vi "DAC Init Results.vi"(8 "error in":errorcluster, 9 "Log Details?":bool, 10 "tdms file":refnum<k34>, 11 "DAC Vacum Valve in":refnum<class "DAC Vacum Valve.lvclass">) -> (0 "error out":errorcluster, 2 "tdms file out":refnum<k34>)   [LabVIEW 2019, in "DAC.lvlib" / "DAC Vacum Valve.lvclass"]
uses:
  DAC Vacum Valve.lvclass
  C:/Users/krio/Documents/LV_Projects/test-stand/App/DAC/DAC.lvclass
  DAC.lvclass/DAC.ctl
  DAC Vacum Valve.lvclass/DAC Vacum Valve.ctl
  DAC.lvclass
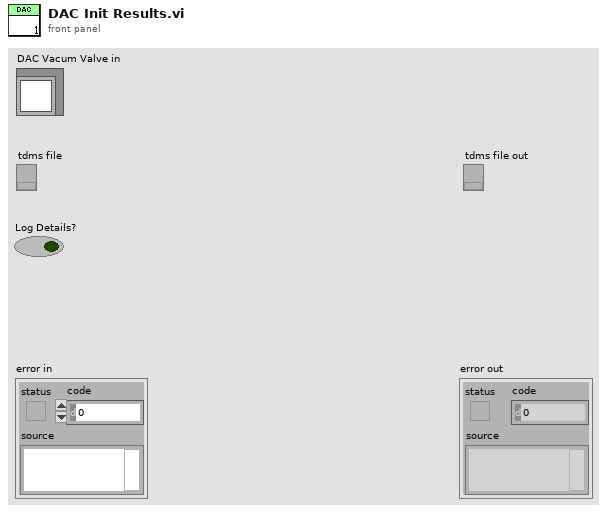
[diagram p1: front panel]
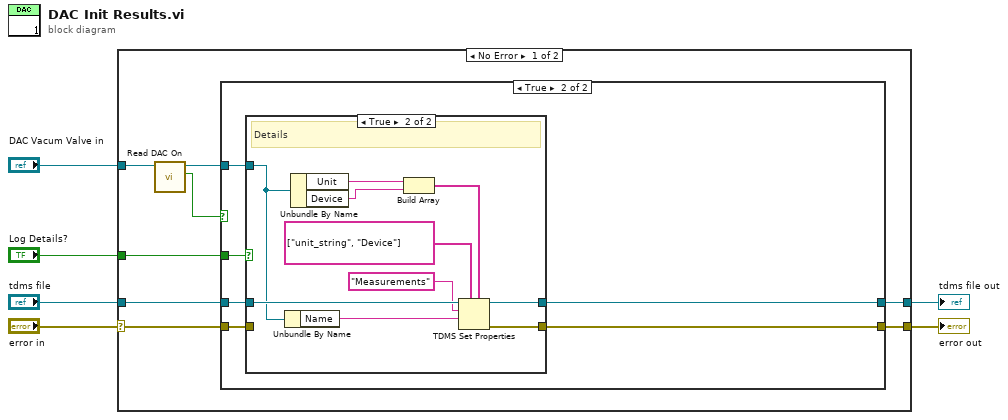
[diagram p0: block diagram]
diagram:
  n1 = case shown="No Error" "error in" {
    selector: "error in" -> [w10 w36]
    tunnel: [w7 w36] -> w6
    tunnel: "DAC Vacum Valve in" -> [w14 _]
    tunnel: "tdms file" -> [w11 w35]
    tunnel: [w8 w35] -> w5
    tunnel: "Log Details?" -> [w9 _]
    frame No Error {
      n2 = call "Read DAC On.vi"("DAC in"=w14) -> ("DAC On"=w12:bool, "DAC out"=w13:refnum<class "DAC Vacum Valve.lvclass">)  [unwired: 8 in, 1 out]
      n3 = case shown="True" w12 {
        tunnel: w11 -> [w15 w22]
        tunnel: [w15 w19] -> w8
        tunnel: [w16 w18] -> w7
        tunnel: w13 -> [_ w21]
        tunnel: w10 -> [w16 w17]
        tunnel: w9 -> [_ w20]
        frame False {
        }
        frame True {
          n4 = case shown="True" w20 {
            tunnel: w22 -> [w24 w34]
            tunnel: [w24 w29] -> w19
            tunnel: [w23 w28] -> w18
            tunnel: w21 -> [_ w25]
            tunnel: w17 -> [w23 _]
            frame False {
            }
            frame True {
              # "Details"
              n5 = Unbundle By Name(w25) -> ("Name"=w27:string)
              n6 = Unbundle By Name(w25) -> ("Unit"=w31:string, "Device"=w26:string)
              n7 = Build Array(w31, w26) -> (w30:string[])
              n8 = TDMS Set Properties(5:w30, 7:string[] ["unit_string", "Device"] ("property names"), 9:w27, 10:"Measurements" ("group name in (Untitled)"), 11:w34) -> (0:w28:errorcluster, 3:w29:refnum<k34>)  [unwired: 1 in, 2 out]
            }
          }
        }
      }
    }
    frame Error {
    }
  }
  "error out" <- w6
  "tdms file out" <- w5
